vi "Build LN2-Scale.vi"() -> ()   [LabVIEW 2019]
uses:
  <userlib>/LevyLab/Build Support/PostBuildSupport/PostBuildSupport.lvclass
  <vilib>/MakerHub/Toolbox/LMH-Toolbox.lvlib
panel:
  in  "Output Package File Path":path=path "C:/Users/patrick/Documents/GitHub/LN2-DIGITAL-SCALE/builds/package/temp.txt"
  in  "Product Name":string="LN2-DIGITAL-SCALE"
  in  "Package Version":string="0.1.1.10"
  in  "Package Source Folder":path=path "C:/Users/patrick/Documents/GitHub/LN2-DIGITAL-SCALE/lvsrc"
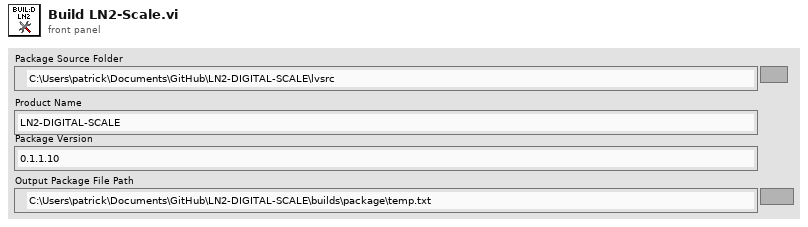
[diagram p1: front panel]
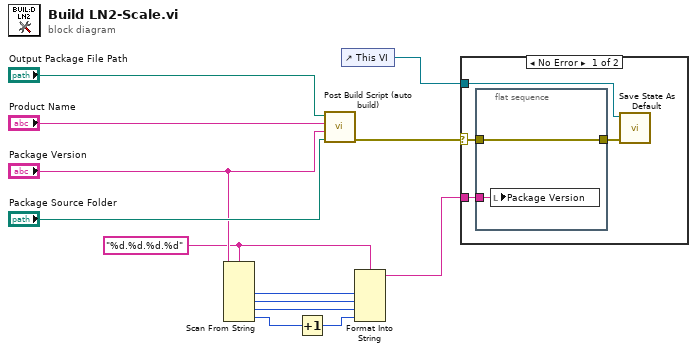
[diagram p0: block diagram]
diagram:
  w8 = "%d.%d.%d.%d" ("format string")
  n1 = Scan From String(format string=w8, input string="Package Version") -> (output 1=w7:i32, output 2=w6:i32, output 3=w1:i32, output 4=w5:i32)  [unwired: 6 in, 3 out]
  n2 = Increment(x=w5) -> (x+1=w4:i32)
  n3 = call <userlib>:"Post Build Script (auto build).vi"("Package Source Folder"="Package Source Folder", "Package Version"="Package Version", "Product Name"="Product Name", "Output Package File Path"="Output Package File Path") -> ("error out"=w10:errorcluster)  [unwired: 7 in]
  n4 = control-ref of="This VI"() -> (w2:refnum<vi>)
  n5 = Format Into String(format string=w8, w7, w6, w1, w4) -> (resulting string=w3:string)  [unwired: 2 in, 1 out]
  n6 = case shown="No Error" w10 {
    selector: w10 -> [w16 _]
    tunnel: w3 -> [w17 _]
    tunnel: w2 -> [w14 _]
    frame No Error {
      n7 = flat-sequence {
        tunnel: w17 -> [w19]
        tunnel: w16 -> [w18]
        tunnel: [w18] -> w15
        frame #0 {
          n8 = local write "Package Version"(w19) -> ()
        }
      }
      n9 = call <vilib>:"Save State As Default.vi"("Error In"=w15, "Target VI"=w14) -> ()  [unwired: 8 in, 2 out]
    }
    frame Error {
    }
  }
